vi "convert motion step with u8 positions to u16.vi"(8 "error in":errorcluster, 10 "data string":string, 11 "Motion Data Cluster in":T1={"Power Supply Voltage"=0.0, "Min Avg Current"=0.0, "Max Avg Current"=0.0, "Min Run Time"=0.0, "Max Run Time"=0.0, "Min Speed"=0.0, "Max Speed"=0.0, "AP Data % of Threshold"=0.0, "Travel Distance"=0.0, "AP Data Type"=enum."91/61", "Check Current"=FALSE, "Check Run Time"=FALSE, "Check Speed"=FALSE, "Express Motion?"=FALSE, "Check Sound Test"=FALSE, "Check Position?"=FALSE, "Collect AP Data"=FALSE, "Inital Position"=0, "End Position"=0, "Goto Posiition"=0, "Max max Current"=0.0, "Min max Current"=0.0, "Check max Current"=FALSE, "Check Sound"=FALSE, "Min Sound (dB)"=0.0, "Max Sound (dB)"=0.0, "SW Mode"=enum."Hard Switch", "LIN Msg"={"ID"=0, "Msg"=[], "LDF"="EX1H"}} {"LIN Msg"."Msg" format="%02x"; "LIN Msg"."ID" format="%02x"}) -> (0 "error out":errorcluster, 3 "Motion Data Cluster out":T1={"Power Supply Voltage"=0.0, "Min Avg Current"=0.0, "Max Avg Current"=0.0, "Min Run Time"=0.0, "Max Run Time"=0.0, "Min Speed"=0.0, "Max Speed"=0.0, "AP Data % of Threshold"=0.0, "Travel Distance"=0.0, "AP Data Type"=enum."91/61", "Check Current"=FALSE, "Check Run Time"=FALSE, "Check Speed"=FALSE, "Express Motion?"=FALSE, "Check Sound Test"=FALSE, "Check Position?"=FALSE, "Collect AP Data"=FALSE, "Inital Position"=0, "End Position"=0, "Goto Posiition"=0, "Max max Current"=0.0, "Min max Current"=0.0, "Check max Current"=FALSE, "Check Sound"=FALSE, "Min Sound (dB)"=0.0, "Max Sound (dB)"=0.0, "SW Mode"=enum."Hard Switch", "LIN Msg"={"ID"=0, "Msg"=[], "LDF"="EX1H"}} {"LIN Msg"."Msg" format="%02x"; "LIN Msg"."ID" format="%02x"})   [LabVIEW 2018]
uses:
  type defs/17x Audit Motion Data Seq Control.ctl
  type defs/17x AP Data Type.ctl
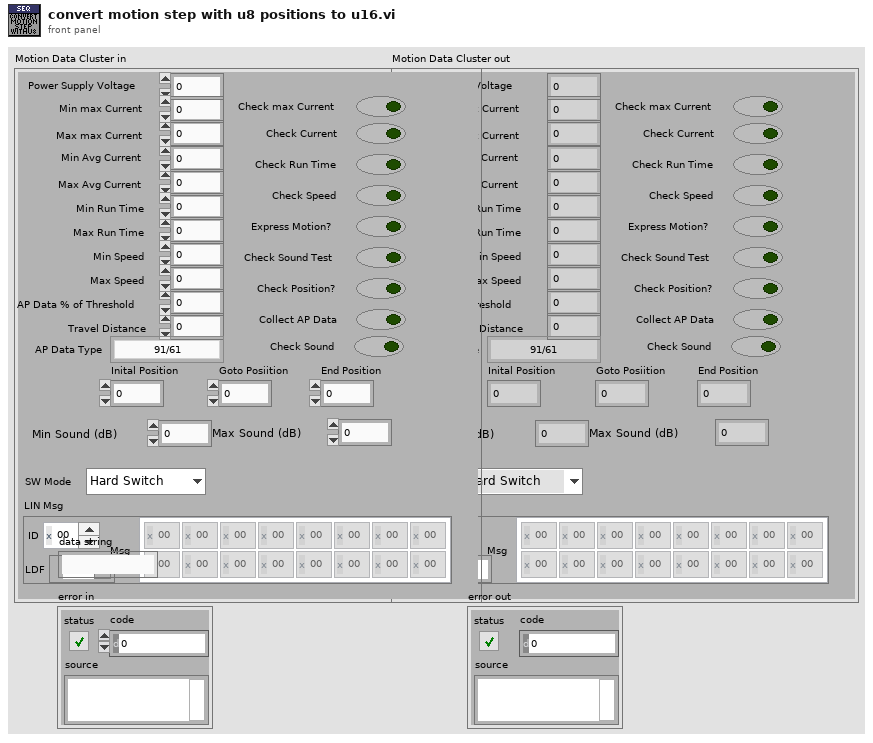
[diagram p1: front panel]
types:
  T1 = typedef "17x Audit Motion Data Seq Control.ctl" = cluster{"Power Supply Voltage":dbl, "Min Avg Current":dbl, "Max Avg Current":dbl, "Min Run Time":dbl, "Max Run Time":dbl, "Min Speed":dbl, "Max Speed":dbl, "AP Data % of Threshold":dbl, "Travel Distance":dbl, "AP Data Type":T2, "Check Current":bool, "Check Run Time":bool, "Check Speed":bool, "Express Motion?":bool, "Check Sound Test":bool, "Check Position?":bool, "Collect AP Data":bool, "Inital Position":u16, "End Position":u16, "Goto Posiition":u16, "Max max Current":dbl, "Min max Current":dbl, "Check max Current":bool, "Check Sound":bool, "Min Sound (dB)":dbl, "Max Sound (dB)":dbl, "SW Mode":enum16{"Hard Switch", "Uncond Frame"}, "LIN Msg":cluster{"ID":u8, "Msg":u8[][], "LDF":refnum<k21>}}
  T2 = typedef "17x AP Data Type.ctl" = enum16{"91/61", "92/62", "93/63", "67", "68", "6F", "71", "91 Msg", "92 Msg", "93 Msg", "94 Msg", "HiRain 91", "HiRain 92 Speed", "HiRain 92 HS", "HiRain 92", "HiRain 93", "SnT"}
  T3 = cluster{"Power Supply Voltage":dbl, "Min Avg Current":dbl, "Max Avg Current":dbl, "Min Run Time":dbl, "Max Run Time":dbl, "Min Speed":dbl, "Max Speed":dbl, "AP Data % of Threshold":dbl, "Travel Distance":dbl, "AP Data Type":T2, "Check Current":bool, "Check Run Time":bool, "Check Speed":bool, "Express Motion?":bool, "Check Sound Test":bool, "Check Position?":bool, "Collect AP Data":bool, "Inital Position":u8, "End Position":u8, "Goto Posiition":u16, "Check max Current":bool, "Max max Current":dbl, "Min max Current":dbl}
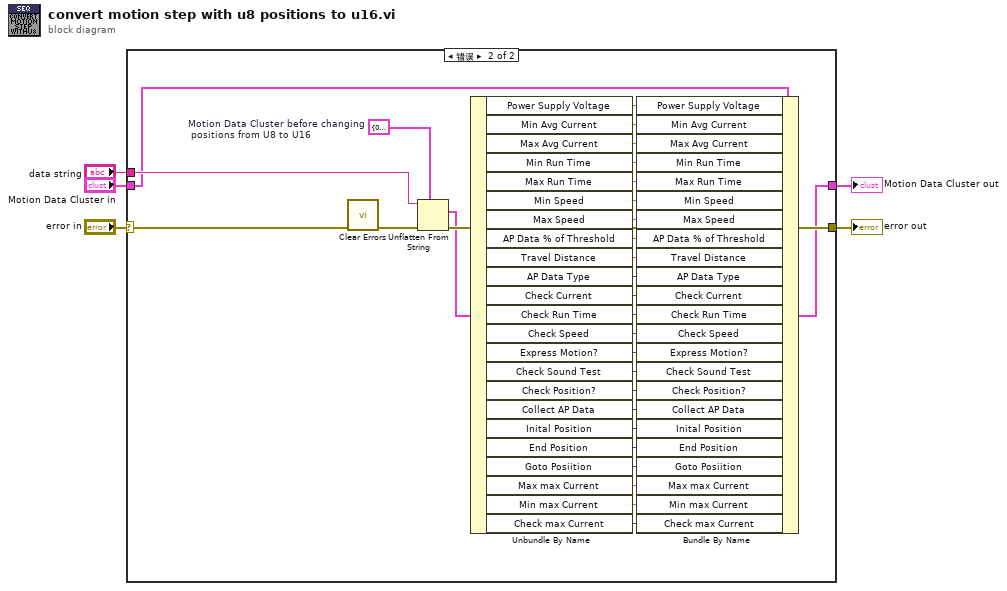
[diagram p0: block diagram]
diagram:
  n1 = case shown="错误" "error in" {
    selector: "error in" -> [w7 w37]
    tunnel: [w7 w34] -> w2
    tunnel: "data string" -> [_ w35]
    tunnel: "Motion Data Cluster in" -> [w6 w32]
    tunnel: [w6 w11] -> w5
    frame No Error {
    }
    frame Error {
      w36 = T3 {"Power Supply Voltage"=0.0, "Min Avg Current"=0.0, "Max Avg Current"=0.0, "Min Run Time"=0.0, "Max Run Time"=0.0, "Min Speed"=0.0, "Max Speed"=0.0, "AP Data % of Threshold"=0.0, "Travel Distance"=0.0, "AP Data Type"=enum."91/61", "Check Current"=FALSE, "Check Run Time"=FALSE, "Check Speed"=FALSE, "Express Motion?"=FALSE, "Check Sound Test"=FALSE, "Check Position?"=FALSE, "Collect AP Data"=FALSE, "Inital Position"=0, "End Position"=0, "Goto Posiition"=0, "Check max Current"=FALSE, "Max max Current"=0.0, "Min max Current"=0.0}  # Motion Data Cluster before changing  positions from U8 to U16
      n2 = call <vilib>:"Clear Errors.vi"("error in (no error)"=w37) -> ("error out"=w38:errorcluster)  [unwired: 5 in, 1 out]
      n3 = Unflatten From String(type=w36, binary string=w35, error in (no error)=w38) -> (value=w33:T3, error out=w34:errorcluster)  [unwired: 2 in, 1 out]
      n4 = Unbundle By Name(w33) -> ("Power Supply Voltage"=w31:dbl, "Min Avg Current"=w30:dbl, "Max Avg Current"=w29:dbl, "Min Run Time"=w28:dbl, "Max Run Time"=w27:dbl, "Min Speed"=w26:dbl, "Max Speed"=w25:dbl, "AP Data % of Threshold"=w24:dbl, "Travel Distance"=w23:dbl, "AP Data Type"=w22:T2, "Check Current"=w21:bool, "Check Run Time"=w20:bool, "Check Speed"=w19:bool, "Express Motion?"=w18:bool, "Check Sound Test"=w17:bool, "Check Position?"=w16:bool, "Collect AP Data"=w15:bool, "Inital Position"=w14:u8, "End Position"=w13:u8, "Goto Posiition"=w12:u16, "Max max Current"=w8:dbl, "Min max Current"=w9:dbl, "Check max Current"=w10:bool)
      n5 = Bundle By Name(cluster=w32, "Power Supply Voltage"=w31, "Min Avg Current"=w30, "Max Avg Current"=w29, "Min Run Time"=w28, "Max Run Time"=w27, "Min Speed"=w26, "Max Speed"=w25, "AP Data % of Threshold"=w24, "Travel Distance"=w23, "AP Data Type"=w22, "Check Current"=w21, "Check Run Time"=w20, "Check Speed"=w19, "Express Motion?"=w18, "Check Sound Test"=w17, "Check Position?"=w16, "Collect AP Data"=w15, "Inital Position"=w14, "End Position"=w13, "Goto Posiition"=w12, "Max max Current"=w8, "Min max Current"=w9, "Check max Current"=w10) -> (w11:T1)
    }
  }
  "Motion Data Cluster out" <- w5
  "error out" <- w2
